vi "Fill Error Details.vi"(8 "error in":errorcluster, 10 "call stack index":i32, 11 "error code":i32) -> (0 "error out":errorcluster)   [LabVIEW 2020, in "AIM ARINC 429 Hardware API.lvlib"]
uses:
  AIM ARINC 429 Hardware API.lvlib
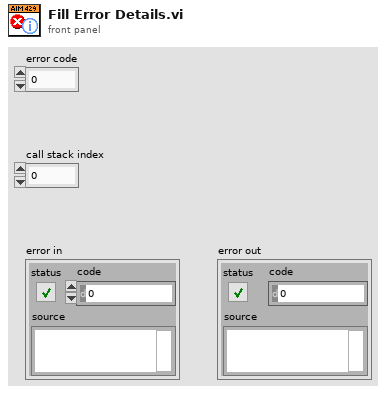
[diagram p1: front panel]
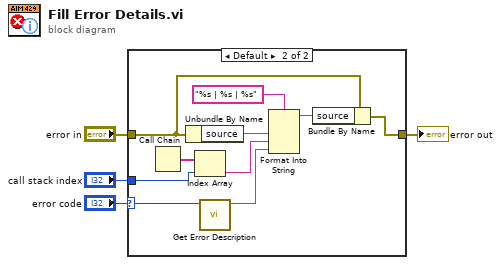
[diagram p0: block diagram]
diagram:
  n1 = case shown="Default" "error code" {
    selector: "error code" -> [_ w11]
    tunnel: "error in" -> [w5 w10]
    tunnel: [w5 w9] -> w4
    tunnel: "call stack index" -> [_ w6]
    frame 0 {
    }
    frame Default {
      n2 = Call Chain() -> (call chain=w15:string[])
      n3 = Unbundle By Name(w10) -> ("source"=w8:string)
      n4 = Index Array(array=w15, index=w6) -> (element=w13:string)
      n5 = call "Get Error Description.vi"("error code"=w11) -> ("error description"=w12:string)  [unwired: 9 in, 1 out]
      n6 = Format Into String(format string="%s | %s | %s", w8, w13, w12) -> (resulting string=w7:string)  [unwired: 2 in, 1 out]
      n7 = Bundle By Name(cluster=w10, "source"=w7) -> (w9:errorcluster)
    }
  }
  "error out" <- w4
